vi "Read IPS PSU Field remove.vi"(6 "Axis":T1, 8 "error in (no error)":errorcluster, 11 "Instrument.OxfordVRM in":refnum<class "Instrument.OxfordVRM.lvclass">) -> (0 "error out":errorcluster, 2 "Power Supply Field (T)":dbl, 3 "Instrument.OxfordVRM out":refnum<class "Instrument.OxfordVRM.lvclass">)   [LabVIEW 2016, in "Instrument.OxfordVRM.lvclass"]
uses:
  Instrument.OxfordVRM.lvclass
  <userlib>/LevyLab/Levylab Instruments/Instrument Types/Cryostat/Typedefs/Magnet Axis--Enum.ctl
  Instrument.OxfordVRM.lvclass/Instrument.OxfordVRM.ctl
  <instrlib>/Mercury iXX/Public/Libraries/Magnet/Open/Open Magnet Device.vi
  <instrlib>/Mercury iXX/Public/Libraries/Magnet/Signals/Read/Field (Read).vi
  <instrlib>/Mercury iXX/Mercury iXX.lvlib
  <instrlib>/Mercury iXX/Public/Libraries/Magnet.lvlib
  <userlib>/LevyLab/Levylab Instruments/Instrument Types/Cryostat/Instrument.Cryostat.lvclass
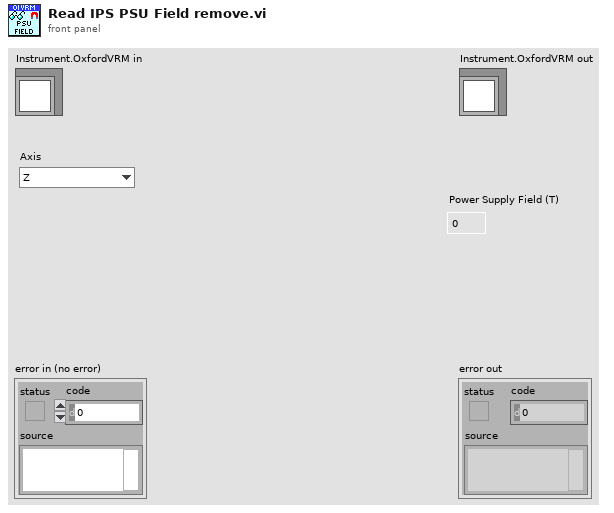
[diagram p1: front panel]
types:
  T1 = typedef "Instrument.Cryostat.lvclass/Magnet Axis--Enum.ctl" = enum16{"Z", "X", "Y"}
  T2 = typedef "Mercury iXX.lvlib/Mercury Reference.ctl" = cluster{"Comms":refnum<visa-resource-name>, "Device ID":string[], "Comms Layer":T3, "Command":string, "Query reference":T4}
  T3 = typedef "Mercury iXX.lvlib/Comms Transport Layer.ctl" = enum16{"Ethernet TCP/IP", "USB", "ISOBus - RS-232", "GPIB"}
  T4 = typedef "Mercury iXX.lvlib/Query Dynamic Reference.ctl" = refnum<vi>
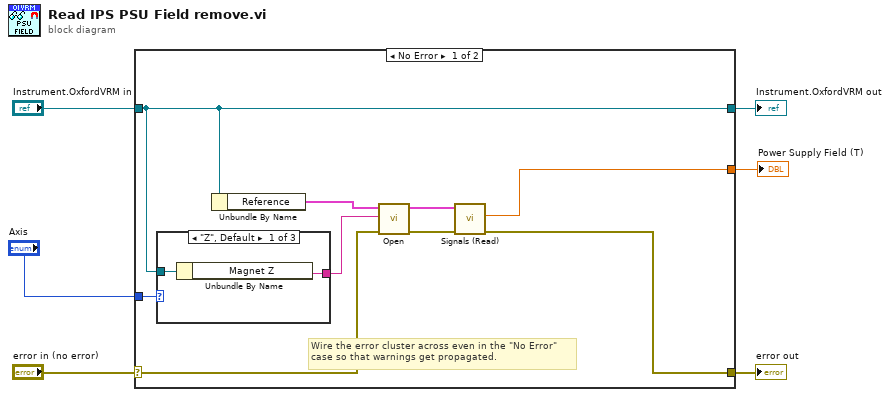
[diagram p0: block diagram]
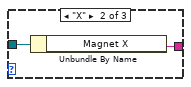
[diagram p2: hidden frame]
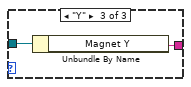
[diagram p3: hidden frame]
diagram:
  n1 = case shown="No Error" "error in (no error)" {
    selector: "error in (no error)" -> [w12 w23]
    tunnel: [w11 w23] -> w5
    tunnel: [w8 w22] -> w3
    tunnel: "Instrument.OxfordVRM in" -> [w8 w22]
    tunnel: [w10 _] -> w2
    tunnel: "Axis" -> [w9 _]
    frame No Error {
      # "Wire the error cluster across even in the \"No Error\"\ncase so that warnings get propagated."
      n2 = case shown="\"Z\", Default" w9 {
        tunnel: [w17 w19 w20] -> w7
        tunnel: w8 -> [w16 w18 w21]
        frame "Z", Default {
          n3 = Unbundle By Name(w16) -> ("Magnet Z"=w17:string)
        }
        frame "X" {
          n4 = Unbundle By Name(w18) -> ("Magnet X"=w19:string)
        }
        frame "Y" {
          n5 = Unbundle By Name(w21) -> ("Magnet Y"=w20:string)
        }
      }
      n6 = Unbundle By Name(w8) -> ("Reference"=w13:T2)
      n7 = call-poly <instrlib>:"Open.vi"("error in (no error)"=w12, "Device Identifier"=w7, "Mercury Reference In"=w13) -> ("error out"=w15:errorcluster, "Mercury Reference Out"=w14:T2)  [unwired: 7 out]
      n8 = call-poly <instrlib>:"Signals (Read).vi"("error in"=w15, "Mercury Reference In"=w14) -> ("error out"=w11:errorcluster, "Field"=w10:dbl)  [unwired: 1 in, 7 out]
    }
    frame Error {
    }
  }
  "error out" <- w5
  "Instrument.OxfordVRM out" <- w3
  "Power Supply Field (T)" <- w2
